vi "Split Sequences.vi"(8 "error in (no error)":errorcluster, 11 "Scheduler in":refnum<class "Scheduler.lvclass">=refnum) -> (0 "error out":errorcluster, 3 "Scheduler out":refnum<class "Scheduler.lvclass">)   [LabVIEW 2020, in "CIRCUS_uServices.lvlib" / "Scheduler.lvlib" / "Scheduler.lvclass"]
uses:
  Scheduler.lvclass
  Run Utilities/Sequence of SBlocks/Sequence of SBlocks.lvclass
  TALOS/TALOS_PPL.lvlibp
  C:/Users/marco/Documents/GitHub_Lab/CIRCUS/TALOS/TALOS_PPL.lvlibp/Father of all uServices/Father of all uServices/Father of all uServices.lvclass
  C:/Users/marco/Documents/GitHub_Lab/CIRCUS/TALOS/TALOS_PPL.lvlibp/Ancestor/Ancestor/Ancestor.lvclass
  C:/Users/marco/Documents/GitHub_Lab/CIRCUS/TALOS/Actor Framework.lvlibp/1abvi3w/vi.lib/ActorFramework/Actor/Actor.lvclass
  C:/Users/marco/Documents/GitHub_Lab/CIRCUS/CIRCUS uServices et al/Scheduler/Scheduler.lvclass
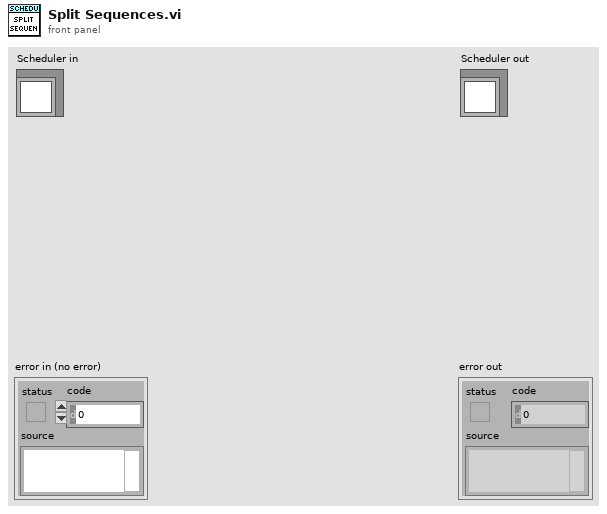
[diagram p1: front panel]
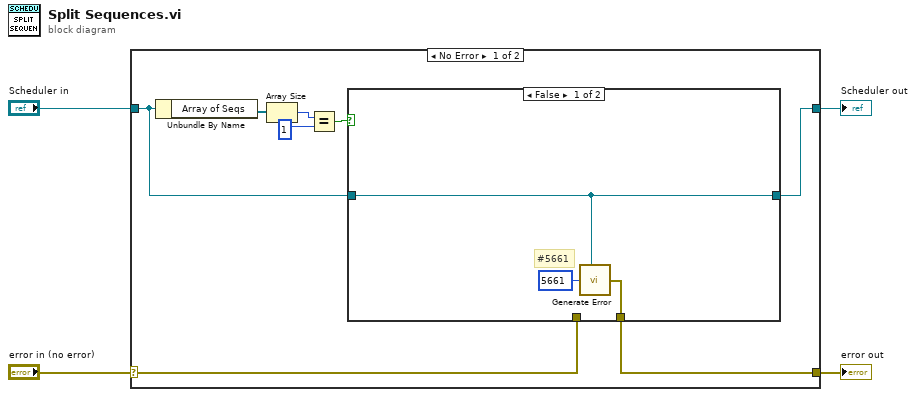
[diagram p0: block diagram]
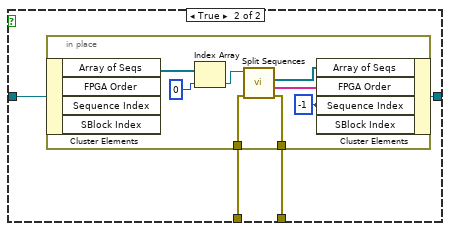
[diagram p2: hidden frame]
diagram:
  n1 = case shown="No Error" "error in (no error)" {
    selector: "error in (no error)" -> [w5 w29]
    tunnel: [w6 w29] -> w3
    tunnel: [w12 w28] -> w1
    tunnel: "Scheduler in" -> [w11 w28]
    frame No Error {
      n2 = Unbundle By Name(w11) -> ("Array of Seqs"=w10:refnum<class "Sequence of SBlocks.lvclass">[])
      n3 = Array Size(array=w10) -> (size(s)=w9:i32)
      n4 = Equal?(x=w9, y=1) -> (x = y?=w7:bool)
      n5 = case shown="False" w7 {
        tunnel: [w15 w19] -> w12
        tunnel: w11 -> [w15 w18]
        tunnel: [w14 w17] -> w6
        tunnel: w5 -> [_ w16]
        frame False {
          # "#5661"
          n6 = call "Generate Error.vi"("Class"=w15, "Error Code"=5661) -> ("error out"=w14:errorcluster)  [unwired: 5 in]
        }
        frame True {
          n7 = in-place {
            in-place-border: [w21] -> w17
            in-place-border: w16 -> [w20]
            w27 = -1 ("Sequence Index")
            n8 = in-place-cluster #1(w18) -> ("Array of Seqs"=w26:refnum<class "Sequence of SBlocks.lvclass">[])  [unwired: 3 out]
            n9 = Index Array(array=w26, index=0) -> (element=w22:refnum<class "Sequence of SBlocks.lvclass">)
            n10 = call "Split Sequences.vi"("error in (no error)"=w20, "Sequence of SBlocks in"=w22) -> ("error out"=w21:errorcluster, "Kasli Order"=w24:string[], "Array of Sequences"=w23:refnum<class "Sequence of SBlocks.lvclass">[])  [unwired: 6 in, 1 out]
            n11 = in-place-cluster #1("Array of Seqs"=w23, "FPGA Order"=w24, "Sequence Index"=w27, "SBlock Index"=w27) -> (w19:refnum<class "Scheduler.lvclass">)
          }
        }
      }
    }
    frame Error {
    }
  }
  "error out" <- w3
  "Scheduler out" <- w1
